vi "unflatten gains.vi"(10 "Identifier":string, 11 "Data to Unwrap":string) -> (3 "PID gains":T1 {"proportional gain (Kc)" format="%.2f"; "integral time (Ti, min)" format="%.2f"})   [LabVIEW 2013, in "PID Loop.lvclass"]
uses:
  PID Loop.lvclass
  PID Gains.ctl
  String Parameters.ctl
  <vilib>/NI/Configuration Framework/serializable configuration/NISE_CEF_serializable configuration.lvclass
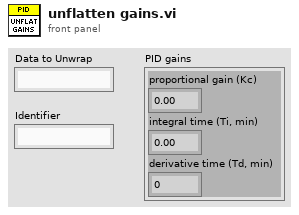
[diagram p1: front panel]
types:
  T1 = typedef "PID Loop.lvclass/PID Gains.ctl" = cluster{"proportional gain (Kc)":dbl, "integral time (Ti, min)":dbl, "derivative time (Td, min)":dbl}
  T2 = typedef "PID Loop.lvclass/String Parameters.ctl" = enum16{"Setpoint", "Process Variable", "Output", "Proportional Gain", "Integral Time", "Derivative Time", "Range High", "Range Low"}
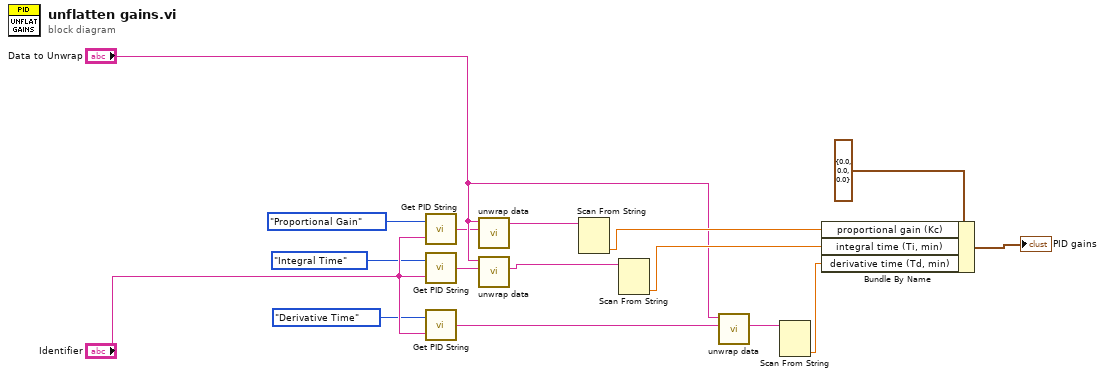
[diagram p0: block diagram]
diagram:
  n1 = call "Get PID String.vi"("PID Loop ID"="Identifier", "PID Parameter"=String_Parameters."Proportional Gain") -> ("Parameter String"=w5:string)
  n2 = call "Get PID String.vi"("PID Loop ID"="Identifier", "PID Parameter"=String_Parameters."Integral Time") -> ("Parameter String"=w4:string)
  n3 = call "Get PID String.vi"("PID Loop ID"="Identifier", "PID Parameter"=String_Parameters."Derivative Time") -> ("Parameter String"=w2:string)
  n4 = call <vilib>:"unwrap data.vi"("identifier"=w5, "data to unwrap"="Data to Unwrap") -> ("unwrapped data"=w10:string)  [unwired: 8 in, 1 out]
  n5 = call <vilib>:"unwrap data.vi"("identifier"=w4, "data to unwrap"="Data to Unwrap") -> ("unwrapped data"=w12:string)  [unwired: 8 in, 1 out]
  n6 = Scan From String(input string=w10) -> (output 1=w11:dbl)  [unwired: 4 in, 3 out]
  n7 = Scan From String(input string=w12) -> (output 1=w13:dbl)  [unwired: 4 in, 3 out]
  n8 = call <vilib>:"unwrap data.vi"("identifier"=w2, "data to unwrap"="Data to Unwrap") -> ("unwrapped data"=w14:string)  [unwired: 8 in, 1 out]
  n9 = Scan From String(input string=w14) -> (output 1=w15:dbl)  [unwired: 4 in, 3 out]
  n10 = Bundle By Name(cluster=T1 {"proportional gain (Kc)"=0.0, "integral time (Ti, min)"=0.0, "derivative time (Td, min)"=0.0} ("PID gains"), "proportional gain (Kc)"=w11, "integral time (Ti, min)"=w13, "derivative time (Td, min)"=w15) -> (→"PID gains":T1)
